vi "ReadLJMconstants.vi"(0 "Selected Register":i32) -> (1 "Nearest Likely Register":i32, 2 "Register Name":string, 3 "Data Type":string)   [LabVIEW 2015]
doc: "In order to Read and Write to any of the numerous pre-configured LabJack T7 Registers, the expected data type needs to be identified. This VI parses the T7 MODBUS Map (.json file), and searches the array to identify the Data Type expected for a desired Register. It also returns the Register Name. Like Registers are grouped in the Map list (e.g. AIN#(0:254)), so if a Selected Register is not exactly matched, a nearest neighbor is sought toward -Inf, and the values of the Nearest Likely Register are returned."
uses:
  <vilib>/regexp/Match Regular Expression.xnode
panel:
  out "index of element":i32
  in  "Tab Control":T1(tab)=enum."Sort & Search Cluster"
  out "text":string
  out "no header":string
  out "no error descriptions":string
  out "result string":string
  out "number of replacements":i32
  out "Array":string[](array[string])
  in  "Register Description":T2(array[cluster])
  out "\"address\"":string[](array[string])
  out "Register":i32[](array[numeric])
  out "\"name\"":string[](array[string])
  out "Reg Name":string[](array[string])
  out "\"type\"":string[](array[string])
  out "Data Type":string[](array[string])
  out "Unsorted Register Description":T2(array[cluster])
  out "Sorted Register Description":T2(array[cluster])
  in  "MODBUS Map Relative Path":path=path "ljm_constants-stripped.json"
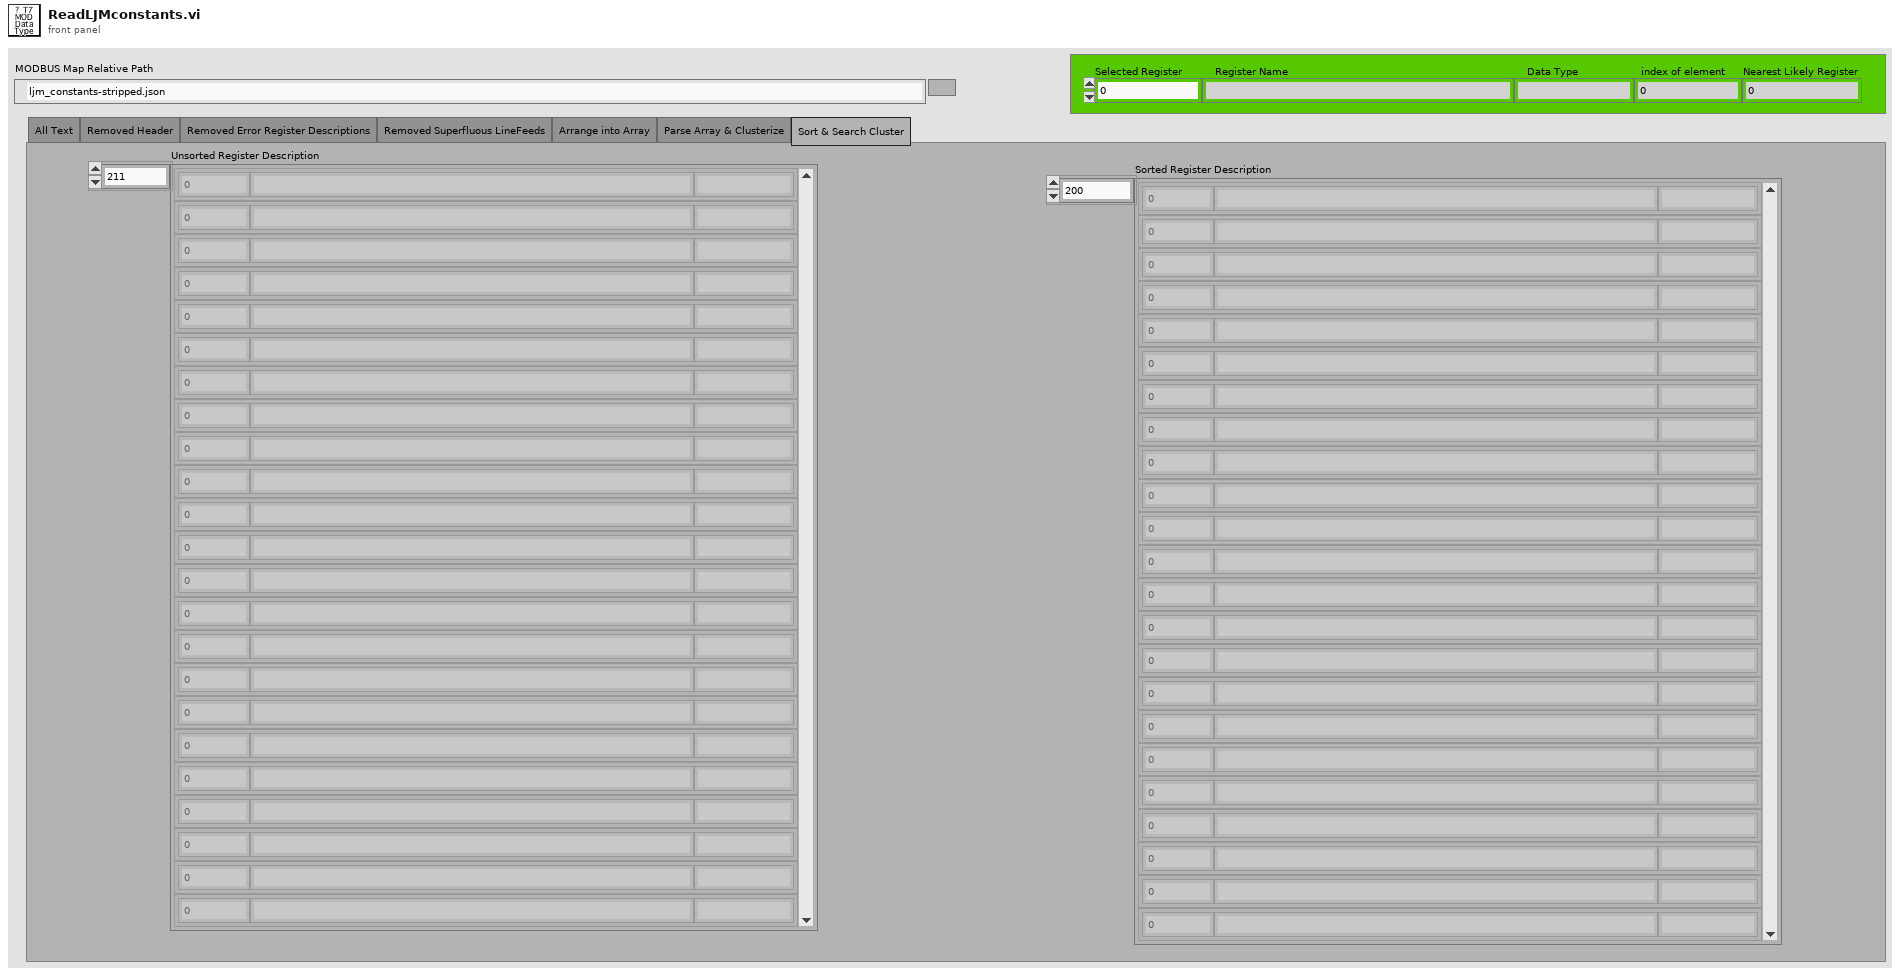
[diagram p1: front panel]
types:
  T1 = enum32{"All Text", "Removed Header", "Removed Error Register Descriptions", "Removed Superfluous LineFeeds", "Arrange into Array", "Parse Array & Clusterize", "Sort & Search Cluster"}
  T2 = cluster{"Register":i32, "Register Name":string, "Data Type":string}[]
  T3 = cluster{"Register":i32, "Register Name":string, "Data Type":string}
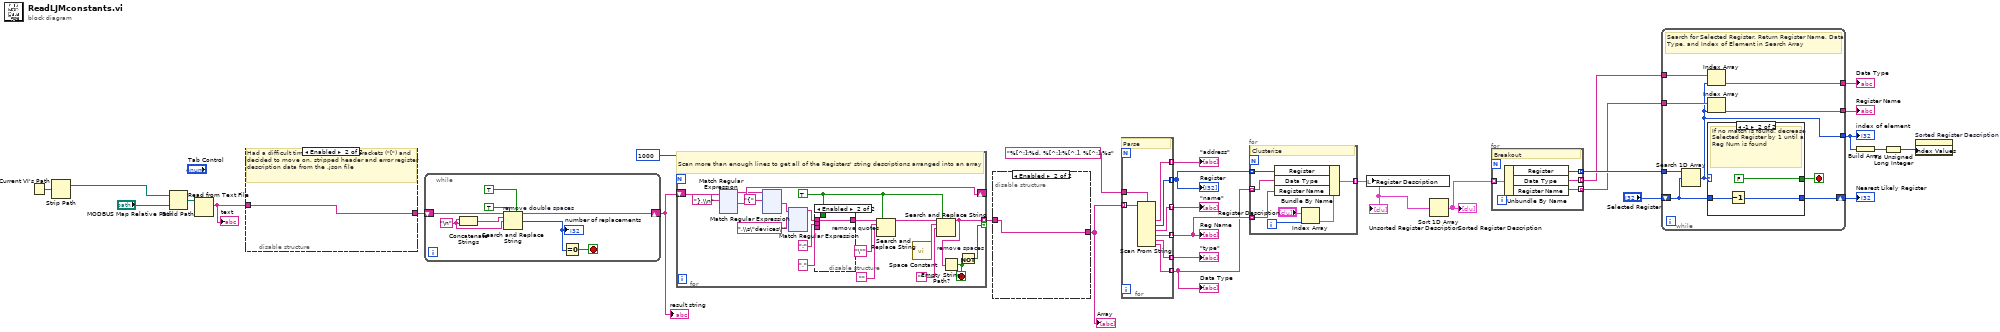
[diagram p0: block diagram]
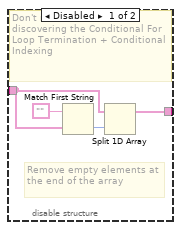
[diagram p2: hidden frame]
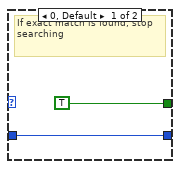
[diagram p3: hidden frame]
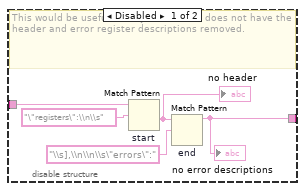
[diagram p4: hidden frame]
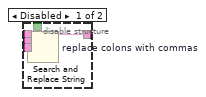
[diagram p5: hidden frame]
diagram:
  n1 = Current VI's Path() -> (path=w4:path)
  n2 = Strip Path(path=w4) -> (stripped path=w3:path)  [unwired: 1 out]
  n3 = Build Path(base path=w3, name or relative path="MODBUS Map Relative Path") -> (appended path=w1:path)
  n4 = Read from Text File(file (use dialog)=w1) -> (text=w29:string)  [unwired: 3 in, 3 out]
  "text" <- w29
  n5 = disable-structure shown="Enabled" {
    disable-tunnel: w29 -> [w34 w35]
    disable-tunnel: [w30 w35] -> w27
    frame Disabled {
      # "This would be useful for a .json file that does not have the header and error register descriptions removed."
      n6 = Match Pattern "start"(string=w34, regular expression="\"registers\":\\n\\s") -> (after substring=w31:string)  [unwired: 4 out]
      "no header" <- w31
      n7 = Match Pattern "end"(string=w31, regular expression="\\s],\\n\\n\\s\"errors\":") -> (before substring=w30:string)  [unwired: 4 out]
      "no error descriptions" <- w30
    }
    frame Enabled {
      # "Had a difficult time parsing around brackets (\"[\") and decided to move on. stripped header and error register description data from the .json file"
    }
  }
  n8 = while {
    shift-right: [w42] -> w26
    shift-left: w27 -> [w43]
    stop <- w36 stop-if-true
    w38 = "\n"
    n9 = Concatenate Strings(w38, w38) -> (w39:string)
    n10 = Search and Replace String "remove double spaces"(replace all?=TRUE ("replace all? (F)"), multiline?=TRUE ("multiline? (F)"), input string=w43, search string=w39, replace string=w38) -> (result string=w42:string, number of replacements=w37:i32)  [unwired: 3 in, 2 out]
    "number of replacements" <- w37
    n11 = Equal To 0?(x=w37) -> (x = 0?=w36:bool)
  }
  "result string" <- w26
  n12 = for {
    N: 1000 -> [_]
    shift-right: [w61] -> _
    shift-left: w26 -> [w63]
    tunnel: [w46] -> w18 mode=indexing if=w44
    stop <- w45 stop-if-true
    w49 = TRUE ("replace all? (F)")
    # "Scan more than enough lines to get all of the Registers' string descriptions arranged into an array"
    n13 = xnode "Match Regular Expression"("input string"=w63, "regular expression"="},\\n") -> ("before match"=w59:string, "after match"=w61:string)  [unwired: 4 in, 3 out]
    n14 = xnode "Match Regular Expression"("input string"=w59, "regular expression"="{") -> ("after match"=w57:string)  [unwired: 4 in, 4 out]
    n15 = xnode "Match Regular Expression"("input string"=w57, "regular expression"=",\\s\"devices\"") -> ("before match"=w56:string)  [unwired: 4 in, 4 out]
    n16 = disable-structure shown="Enabled" {
      disable-tunnel: w56 -> [w68 w69]
      disable-tunnel: ":" ("search string") -> [w67 _]
      disable-tunnel: "," ("replace string (\"\")") -> [w66 _]
      disable-tunnel: [w65 w69] -> w53
      disable-tunnel: w49 -> [w64 _]
      frame Disabled {
        n17 = Search and Replace String "replace colons with commas"(replace all?=w64, input string=w68, search string=w67, replace string=w66) -> (result string=w65:string)  [unwired: 4 in, 3 out]
      }
      frame Enabled {
      }
    }
    n18 = Search and Replace String "remove quotes"(replace all?=w49, input string=w53, search string="\"", replace string="") -> (result string=w50:string)  [unwired: 4 in, 3 out]
    n19 = call <vilib>:"Space Constant.vi"() -> ("String"=w48:string)
    n20 = Search and Replace String "remove spaces"(replace all?=w49, input string=w50, search string=w48, replace string="") -> (result string=w46:string)  [unwired: 4 in, 3 out]
    n21 = Empty String/Path?(string/path=w46) -> (empty?=w45:bool)
    n22 = Not(x=w45) -> (.not. x?=w44:bool)
  }
  n23 = disable-structure shown="Enabled" {
    disable-tunnel: w18 -> [w413 w416]
    disable-tunnel: [w412 w416] -> w17
    frame Disabled {
      # "Remove empty elements at the end of the array"
      # "Don't need this since discovering the Conditional For Loop Termination + Conditional Indexing"
      n24 = Match First String(2:w413, 3:"") -> (0:w414:i32)  [unwired: 1 out]
      n25 = Split 1D Array(array=w413, index=w414) -> (first subarray=w412:string[])  [unwired: 1 out]
    }
    frame Enabled {
    }
  }
  "Array" <- w17
  n26 = for {
    tunnel: w17 -> [w424] mode=indexing
    tunnel: "%[^:]:%d, %[^:]:%[^,], %[^:]:%s" ("format string") -> [w423]
    tunnel: [w422] -> w25 mode=indexing
    tunnel: [w421] -> w19 mode=indexing
    tunnel: [w420] -> w24 mode=indexing
    tunnel: [w419] -> w21 mode=indexing
    tunnel: [w418] -> w23 mode=indexing
    tunnel: [w417] -> w20 mode=indexing
    # "Parse"
    n27 = Scan From String(format string=w423, input string=w424) -> (output 1=w422:string, output 2=w421:i32, output 3=w420:string, output 4=w419:string, output 5=w418:string, output 6=w417:string)  [unwired: 2 in, 9 out]
  }
  "\"address\"" <- w25
  "\"name\"" <- w24
  "Reg Name" <- w21
  "\"type\"" <- w23
  "Data Type" <- w20
  "Register" <- w19
  n28 = for {
    tunnel: w19 -> [w431] mode=indexing
    tunnel: w21 -> [w426] mode=indexing
    tunnel: w20 -> [w425] mode=indexing
    tunnel: [w427] -> w16 mode=indexing
    i -> [w429]
    # "Clusterize"
    n29 = Index Array(array="Register Description", index=w429) -> (element=w428:T3)
    n30 = Bundle By Name(cluster=w428, "Register"=w431, "Data Type"=w425, "Register Name"=w426) -> (w427:T3)
  }
  "Unsorted Register Description" <- w16
  n31 = local write "Register Description"(w16) -> ()
  n32 = Sort 1D Array(array=w16) -> (sorted array=w15:T2)
  "Sorted Register Description" <- w15
  n33 = for {
    tunnel: w15 -> [w435] mode=indexing
    tunnel: [w434] -> w13 mode=indexing
    tunnel: [w433] -> w12 mode=indexing
    tunnel: [w432] -> w11 mode=indexing
    # "Breakout"
    n34 = Unbundle By Name(w435) -> ("Register"=w434:i32, "Data Type"=w433:string, "Register Name"=w432:string)
  }
  n35 = while {
    shift-right: [w444] -> w8
    shift-left: "Selected Register" -> [w441]
    tunnel: w13 -> [w442]
    tunnel: w12 -> [w440]
    tunnel: w11 -> [w439]
    tunnel: [w438] -> w10
    tunnel: [w437] -> w9
    tunnel: [w436] -> w7
    stop <- w443 stop-if-true
    # "Search for Selected Register. Return Register Name, Data Type, and Index of Element in Search Array"
    n36 = Search 1D Array(1D array=w442, element=w441) -> (index of element=w436:i32)  [unwired: 1 in]
    n37 = Index Array(array=w440, index=w436) -> (element=w438:string)
    n38 = Index Array(array=w439, index=w436) -> (element=w437:string)
    n39 = case shown="-1" w436 {
      tunnel: w441 -> [w446 w449]
      tunnel: [w446 w448] -> w444
      tunnel: [TRUE FALSE] -> w443
      frame 0, Default {
        # "If exact match is found, stop searching"
      }
      frame -1 {
        # "If no match is found, decrease Selected Register by 1 until a Reg Num is found"
        n40 = Decrement(x=w449) -> (x-1=w448:i32)
      }
    }
  }
  "Data Type" <- w10
  "Register Name" <- w9
  "index of element" <- w7
  "Nearest Likely Register" <- w8
  n41 = Build Array(w7) -> (w6:i32[])
  n42 = To Unsigned Long Integer(number=w6) -> (unsigned 32bit integer=w5:u32[])
  n43 = property on="Sorted Register Description" class="Arr (strict)"("Index Values"=w5) -> ()  [unwired: 2 in, 2 out]
